vi "Self-Test.vi"(8 "error in (no error)":errorcluster {"code" format="%.0x"}, 11 "VISA Resource Name":refnum<visa-resource-name>) -> (0 "error out":errorcluster {"code" format="%.0x"}, 1 "self-test message":string, 2 "self test result":u32 format="%.0x", 3 "VISA Resource Name Out":refnum<visa-resource-name>)   [LabVIEW 2010, in "Tektronix TDS 3000 Series.lvlib"]
doc: "This VI runs the instrument's self test routine and returns the test result(s)."
uses:
  <instrlib>/Tektronix TDS 3000 Series/Tektronix TDS 3000 Series.lvlib
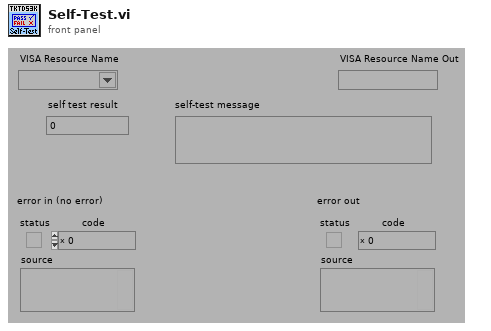
[diagram p1: front panel]
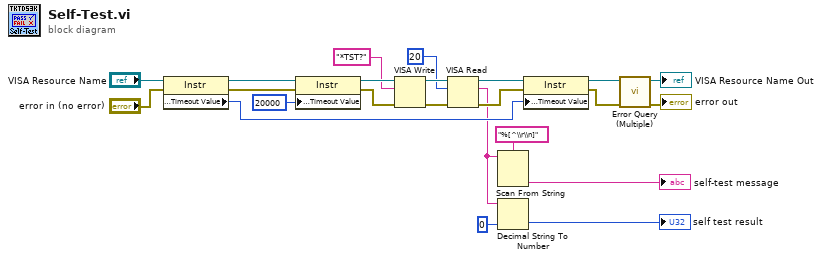
[diagram p0: block diagram]
diagram:
  n1 = property class="Instr"(reference="VISA Resource Name", error in="error in (no error)") -> (reference out=w19:refnum<visa-resource-name>, error out=w20:errorcluster, "General Settings:Timeout Value"=w14:u32)
  n2 = property class="Instr"(reference=w19, error in=w20, "General Settings:Timeout Value"=u32 20000 ("Tmo Value")) -> (reference out=w18:refnum<visa-resource-name>, error out=w17:errorcluster)
  n3 = VISA Write(VISA resource name=w18, write buffer="*TST?" ("Self-Test Command"), error in (no error)=w17) -> (VISA resource name out=w22:refnum<visa-resource-name>, error out=w23:errorcluster)  [unwired: 1 out]
  n4 = VISA Read(VISA resource name=w22, byte count=u32 20 ("byte count (20)"), error in (no error)=w23) -> (VISA resource name out=w15:refnum<visa-resource-name>, read buffer=w10:string, error out=w16:errorcluster)  [unwired: 1 out]
  n5 = Scan From String(format string="%[^\\r\\n]" ("Format String"), input string=w10) -> (output 1=→"self-test message":string)  [unwired: 3 in, 3 out]
  n6 = Decimal String To Number(string=w10, default (0L)=u32 0) -> (number=→"self test result":u32)  [unwired: 1 in, 1 out]
  n7 = property class="Instr"(reference=w15, error in=w16, "General Settings:Timeout Value"=w14) -> (reference out=w4:refnum<visa-resource-name>, error out=w3:errorcluster)
  n8 = call <instrlib>:"Error Query (Multiple).vi"("error in (no error)"=w3, "VISA Resource Name"=w4) -> ("error out"=→"error out":errorcluster, "VISA Resource Name Out"=→"VISA Resource Name Out":refnum<visa-resource-name>)  [unwired: 6 in, 2 out]
